vi "first example.vi"() -> ()   [LabVIEW 2009]
panel:
  in  "endprgm":bool
  out "output":string
  in  "test":bool
  out "nonzero?":bool
  in  "input":dbl
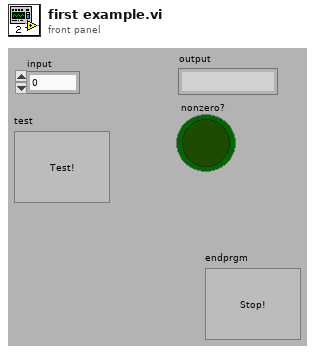
[diagram p1: front panel]
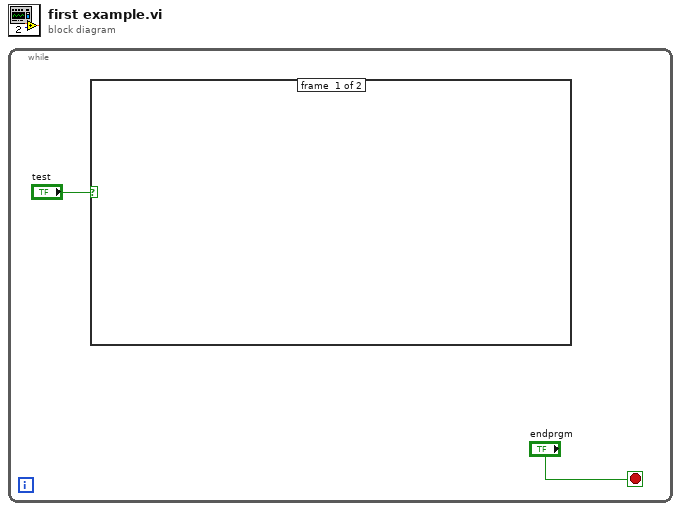
[diagram p0: block diagram]
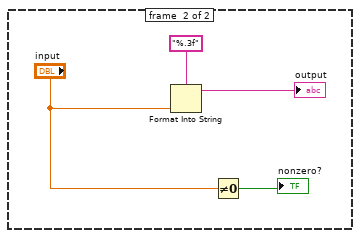
[diagram p2: hidden frame]
diagram:
  n1 = while {
    stop <- "endprgm" stop-if-true
    n2 = case shown="True" "test" {
      frame #0 {
      }
      frame #1 {
        n3 = Format Into String(format string="%.3f", "input") -> (resulting string=→"output":string)  [unwired: 2 in, 1 out]
        n4 = Not Equal To 0?(x="input") -> (x != 0?=→"nonzero?":bool)
      }
    }
  }
